vi "MISCELANEA_WAIT.vi"(4 "ms wait IN":u32=10, 5 "Error IN":errorcluster) -> (18 "ms wait OUT":u32, 19 "Error OUT":errorcluster)   [LabVIEW 2019]
uses:
  Global.Salir Ya.vi
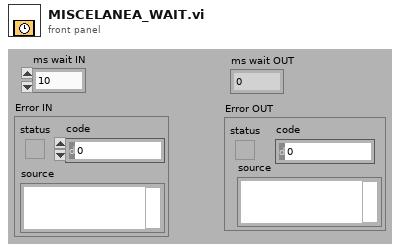
[diagram p1: front panel]
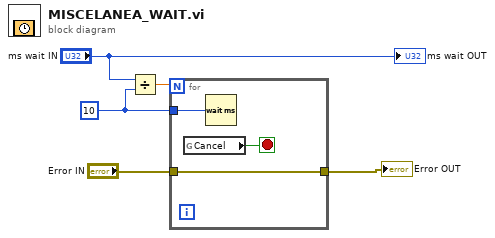
[diagram p0: block diagram]
diagram:
  w4 = u32 10 ("millisecond multiple")
  n1 = Divide(x="ms wait IN", y=w4) -> (x/y=w3:dbl)
  n2 = for {
    N: w3 -> [_]
    tunnel: w4 -> [w8]
    tunnel: [w6] -> w2
    tunnel: "Error IN" -> [w6]
    stop <- w7 stop-if-true
    n3 = global read "Global.Salir Ya.vi" "Cancel"() -> (w7:bool)
    n4 = Wait (ms)(milliseconds to wait=w8) -> ()  [unwired: 1 out]
  }
  "Error OUT" <- w2
  "ms wait OUT" <- "ms wait IN"
